vi "DAQ_Init.vi"(6 "itteration":u16, 9 "Sample time":dbl=0.3) -> (0 "error out":errorcluster, 3 "DAQ Prams":T1={"task in"="", "Num Pts"=14400, "timeout"=2.2, "FIFO"=14400, "Double Bounce"=1.0, "Sensitivity (V/X)"=[]} {"Double Bounce" format="%#.2g"})   [LabVIEW 2022 SP3]
panel:
  out "Sample Rate":u32=48000
  out "Actual Sample Rate":dbl=51200.0 format="%0.2f"
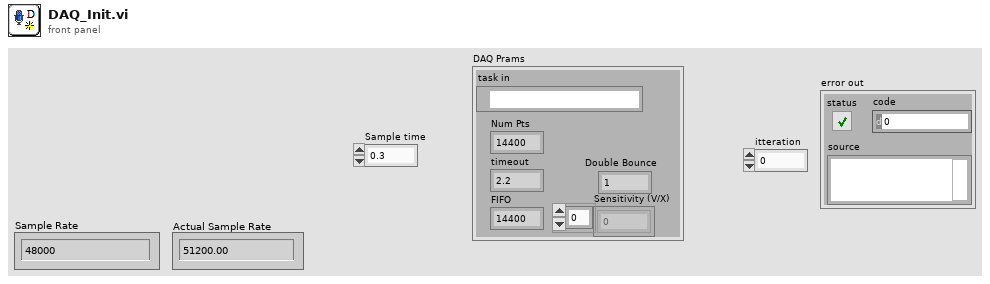
[diagram p1: front panel]
types:
  T1 = cluster{"task in":refnum<k21>, "Num Pts":i32, "timeout":dbl, "FIFO":i32, "Double Bounce":dbl, "Sensitivity (V/X)":dbl[]}
  T2 = cluster{"Sample Clock Source":tag, "Sample Rate":u32, "Hammer":cluster{"Physical Channel":tag, "Terminal Configuration":i32, "IEPE Source":i32, "Current (A)":dbl, "output":u16, "Min Force":dbl, "Max Force":dbl, "Force Sensitivity (mV/N)":dbl}, "Microphone":cluster{"Physical Channel":tag, "Terminal Configuration":i32, "IEPE Source":i32, "Current (A)":dbl, "output":u16, "Min SPL/Acc":dbl, "Max SPL/Acc":dbl, "Sensitivity":dbl}}
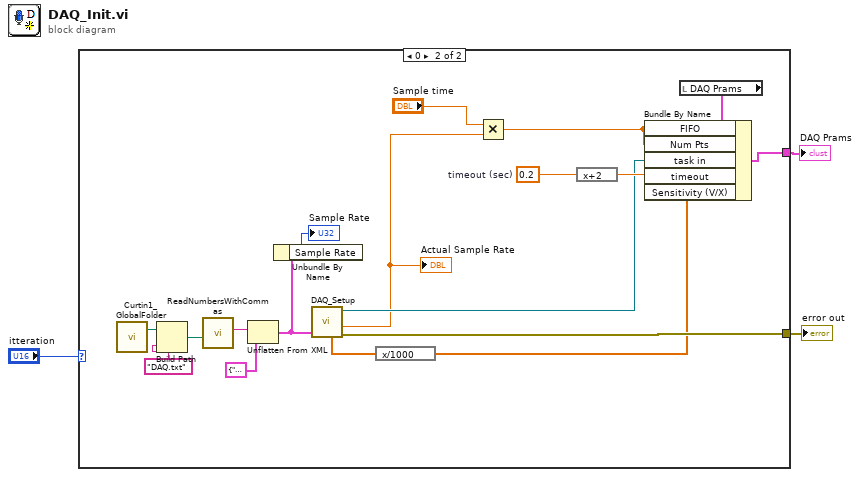
[diagram p0: block diagram]
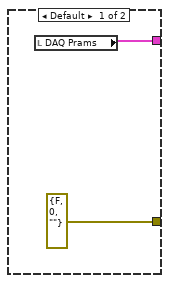
[diagram p2: hidden frame]
diagram:
  n1 = case shown="0" "itteration" {
    tunnel: [w5 w23] -> w3
    tunnel: [errorcluster {"status"=FALSE, "code"=0, "source"=""} ("error out") w17] -> w2
    frame Default {
      n2 = local read "DAQ Prams"() -> (w5:T1)
    }
    frame 0 {
      w11 = 0.2  # timeout (sec)
      n3 = call "Curtin1_GlobalFolder.vi"() -> ("LabVIEW Data Path"=w20:path)  [unwired: 1 in, 1 out]
      n4 = Build Path(base path=w20, name or relative path="DAQ.txt") -> (appended path=w7:path)
      n5 = call "ReadNumbersWithCommas.vi"("file (use dialog)"=w7) -> ("text"=w6:string)  [unwired: 7 in, 3 out]
      n6 = Unflatten From XML(xml string=w6, type=T2 {"Sample Clock Source"="OnboardClock", "Sample Rate"=48000, "Hammer"={"Physical Channel"="Dev2/ai0", "Terminal Configuration"=12529, "IEPE Source"=10200, "Current (A)"=0.004, "output"=0, "Min Force"=-100.0, "Max Force"=100.0, "Force Sensitivity (mV/N)"=50.0}, "Microphone"={"Physical Channel"="Dev2/ai1", "Terminal Configuration"=12529, "IEPE Source"=10200, "Current (A)"=0.004, "output"=0, "Min SPL/Acc"=0.0, "Max SPL/Acc"=120.0, "Sensitivity"=10.0}} ("Params")) -> (value=w15:T2)  [unwired: 1 in, 1 out]
      n7 = Unbundle By Name(w15) -> ("Sample Rate"=→"Sample Rate":u32)
      n8 = call "DAQ_Setup.vi"("Params"=w15) -> ("error out"=w17:errorcluster, "SampClk.Rate"=w13:dbl, "Task out"=w16:refnum<k21>, "Sensitivity (mV/X)"=w9:dbl[])  [unwired: 6 in, 1 out]
      "Actual Sample Rate" <- w13
      n9 = expression code="x/1000"(w9) -> (w8:dbl[])
      n10 = Multiply(x="Sample time", y=w13) -> (x*y=w10:dbl)
      n11 = expression code="x+2"(w11) -> (w21:dbl)
      n12 = local read "DAQ Prams"() -> (w22:T1)
      n13 = Bundle By Name(cluster=w22, "FIFO"=w10, "Num Pts"=w10, "task in"=w16, "timeout"=w21, "Sensitivity (V/X)"=w8) -> (w23:T1)
    }
  }
  "DAQ Prams" <- w3
  "error out" <- w2
